vi "Read Connection Information.vi"(8 "error in (no error)":errorcluster, 11 "ADODB in":refnum<class "ADODB.lvclass">) -> (0 "error out":errorcluster, 2 "Connection Information":path, 3 "ADODB out":refnum<class "ADODB.lvclass">)   [LabVIEW 2020]
uses:
  ADODB.lvclass
  C:/Users/User/Desktop/Raman Program/Database OOP/source/Database OOP/Database/Database Class/Database.lvclass
  C:/Users/User/Desktop/Raman Program/Database OOP/source/Database OOP/Database Advanced Schema/Database Schema.lvclass
  C:/Users/User/Desktop/Raman Program/Database OOP/source/Database OOP/Database Interface/Database Interface.lvclass
  C:/Users/User/Desktop/Raman Program/Database OOP/source/Database OOP/ADODB/ADODB Class/ADODB.lvclass
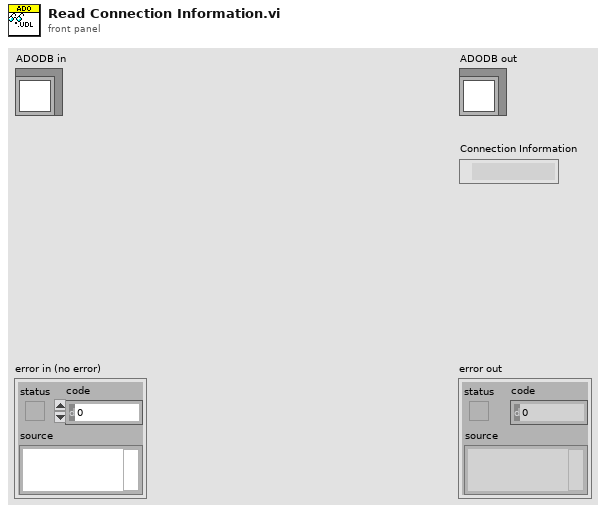
[diagram p1: front panel]
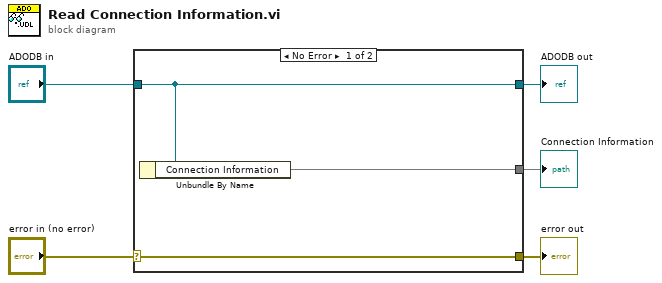
[diagram p0: block diagram]
diagram:
  n1 = case shown="No Error" "error in (no error)" {
    selector: "error in (no error)" -> [w8 w9]
    tunnel: [w8 w9] -> w4
    tunnel: [w7 w10] -> w2
    tunnel: "ADODB in" -> [w7 w10]
    tunnel: [w6 _] -> w1
    frame No Error {
      n2 = Unbundle By Name(w7) -> ("Connection Information"=w6)
    }
    frame Error {
    }
  }
  "error out" <- w4
  "ADODB out" <- w2
  "Connection Information" <- w1
